vi "Example_analog_read_highres.vi"() -> ()   [LabVIEW 2022 SP3]
uses:
  usbtmc_scpi_labtool.lvlib
panel:
  out "Voltage":dbl
  in  "stop":bool
  out "analog out":i32
  in  "Pin":u8 max=7 step=1
  in  "VISA resource name in":refnum<visa-resource-name>="USB0::0xCAFE::0x4000::123456::INSTR"
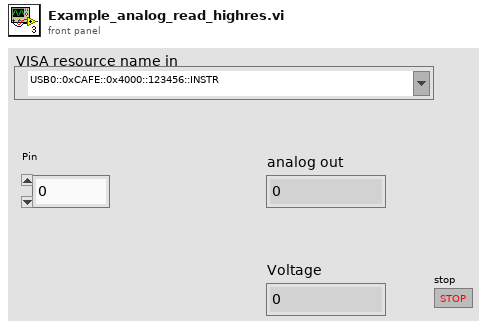
[diagram p1: front panel]
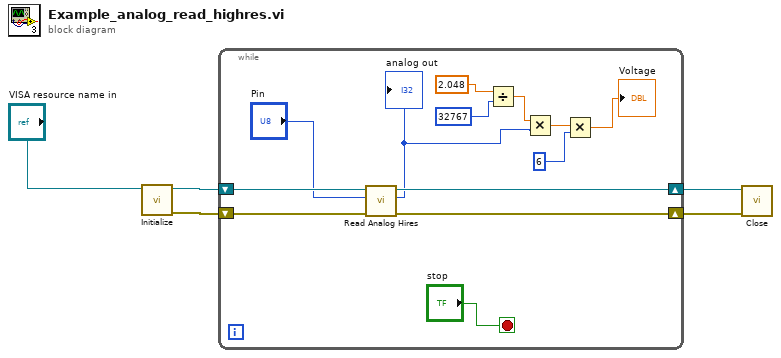
[diagram p0: block diagram]
diagram:
  n1 = call "Initialize.vi"("VISA resource name in"="VISA resource name in") -> ("error out"=w4:errorcluster, "VISA resource name out"=w5:refnum<visa-resource-name>)  [unwired: 9 in]
  n2 = while {
    shift-right: [w16] -> w3
    shift-left: w5 -> [w18]
    shift-right: [w15] -> w2
    shift-left: w4 -> [w17]
    stop <- "stop" stop-if-true
    n3 = call "Read Analog Hires.vi"("error in (no error)"=w17, "Pin"="Pin", "VISA resource name"=w18) -> ("error out"=w15:errorcluster, "analog out"=w9:i32, "VISA resource name out"=w16:refnum<visa-resource-name>)  [unwired: 6 in]
    "analog out" <- w9
    n4 = Divide(x=2.048, y=32767) -> (x/y=w10:dbl)
    n5 = Multiply(x=w10, y=w9) -> (x*y=w8:dbl)
    n6 = Multiply(x=w8, y=6) -> (x*y=→"Voltage":dbl)
  }
  n7 = call "Close.vi"("error in (no error)"=w2, "VISA resource name"=w3) -> ()  [unwired: 10 in]
